vi "Create All Message Queues.vi"(8 "error in (no error)":errorcluster) -> (0 "error out":errorcluster, 3 "Message Queues out":T1)   [LabVIEW 2020, in "Message Queue.lvlib"]
doc: "This VI creates and initializes all the message queues for your application. If your application requires more than one message queue, right-click the \"Message Queues\" constant above and select Open Type Def. Add the new Message Queue(s) to the type definition, then initialize them in this VI."
uses:
  Message Queue.lvlib
  All Message Queues.ctl
  Message Cluster.ctl
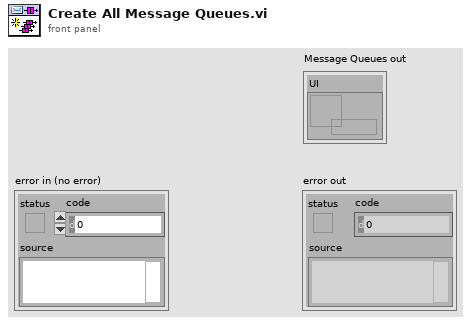
[diagram p1: front panel]
types:
  T1 = typedef "Message Queue.lvlib/All Message Queues.ctl" = cluster{"UI":refnum<queue>}
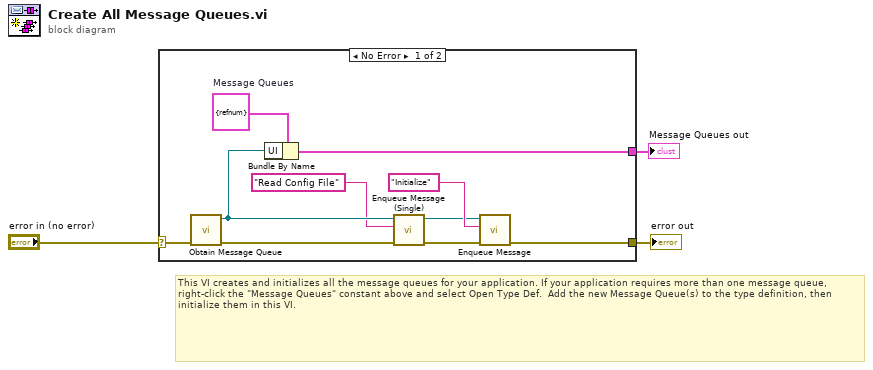
[diagram p0: block diagram]
diagram:
  # "This VI creates and initializes all the message queues for your application. If your application requires more than one message queue, right-click the \"Message Queues\" constant above and select Open Type Def.  Add the new Message Queue(s) to the type definition, then initialize them in this VI."
  n1 = case shown="No Error" "error in (no error)" {
    selector: "error in (no error)" -> [w10 w14]
    tunnel: [w13 w14] -> w3
    tunnel: [w11 _] -> w2
    frame No Error {
      w12 = T1 {"UI"=refnum}  # Message Queues
      n2 = call "Obtain Message Queue.vi"("error in (no error)"=w10) -> ("error out"=w9:errorcluster, "Message Queue"=w5:refnum<queue>)  [unwired: 9 in]
      n3 = Bundle By Name(cluster=w12, "UI"=w5) -> (w11:T1)
      n4 = call "Enqueue Message (Single).vi"("error in (no error)"=w9, "Message"="Read Config File", "Message Queue"=w5) -> ("error out"=w7:errorcluster, "dup Message Queue"=w6:refnum<queue>)  [unwired: 7 in]
      n5 = call-poly "Enqueue Message.vi"("error in (no error)"=w7, "Message"="Initialize", "Message Queue"=w6) -> ("error out"=w13:errorcluster)  [unwired: 7 in, 1 out]
    }
    frame Error {
    }
  }
  "Message Queues out" <- w2
  "error out" <- w3
